vi "Create Progect.vi"(1 "Source DIR":path, 2 "element":string, 3 "selected path":path) -> (0 "Boolean":bool)   [LabVIEW 2019]
panel:
  out "error out":errorcluster
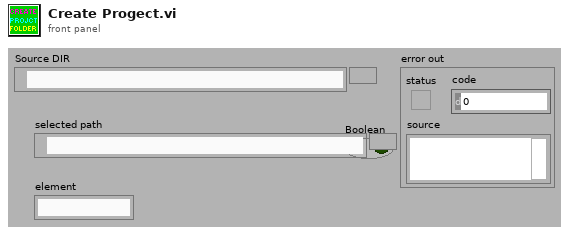
[diagram p1: front panel]
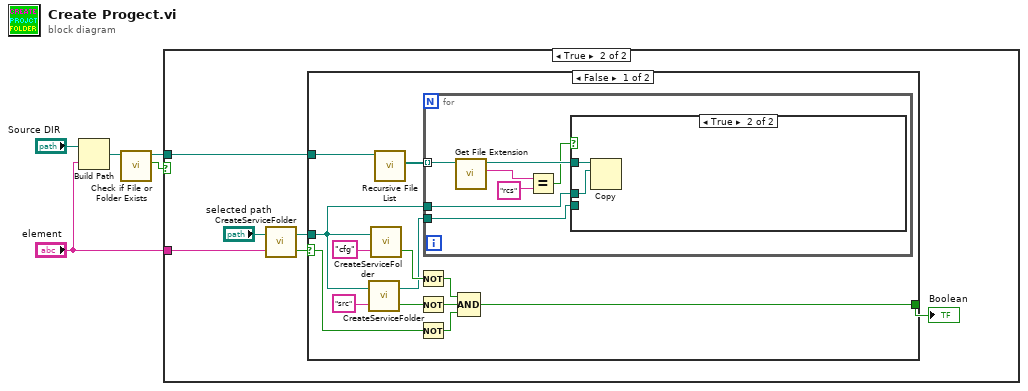
[diagram p0: block diagram]
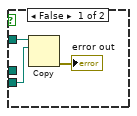
[diagram p3: hidden frame]
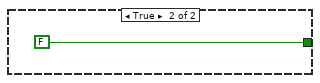
[diagram p4: hidden frame]
diagram:
  n1 = Build Path(base path="Source DIR", name or relative path="element") -> (appended path=w4:path)
  n2 = call <vilib>:"Check if File or Folder Exists.vi"("path"=w4) -> ("file or folder exists?"=w3:bool, "dup path"=w2:path)  [unwired: 8 in, 1 out]
  n3 = case shown="True" w3 {
    tunnel: w2 -> [_ w6]
    tunnel: "element" -> [_ w9]
    frame False {
    }
    frame True {
      n4 = call "CreateServiceFolder.vi"("element"=w9, "selected path"="selected path") -> ("cancelled"=w8:bool, "created path"=w7:path)
      n5 = case shown="False" w8 {
        selector: w8 -> [w21 _]
        tunnel: w7 -> [w12 _]
        tunnel: [w20 FALSE] -> w11
        tunnel: w6 -> [w15 _]
        frame False {
          n6 = call "CreateServiceFolder.vi"("element"="src" ("prompt (Create Folder)"), "selected path"=w12) -> ("cancelled"=w16:bool, "created path"=w13:path)
          n7 = call "CreateServiceFolder.vi"("element"="cfg" ("prompt (Create Folder)"), "selected path"=w12) -> ("cancelled"=w18:bool)  [unwired: 1 out]
          n8 = call <vilib>:"Recursive File List.vi"("Folder Path"=w15) -> ("All Files in Dir"=w14:path[])  [unwired: 6 in, 4 out]
          n9 = Not(x=w18) -> (.not. x?=w24:bool)
          n10 = Not(x=w16) -> (.not. x?=w23:bool)
          n11 = Not(x=w21) -> (.not. x?=w22:bool)
          n12 = for {
            tunnel: w14 -> [w31] mode=indexing
            tunnel: w13 -> [w27]
            tunnel: w12 -> [w26]
            n13 = call <vilib>:"Get File Extension.vi"("file"=w31) -> ("lowercase file extension"=w25:string, "dup file"=w30:path)  [unwired: 6 in, 3 out]
            n14 = Equal?(x=w25, y="rcs" ("lowercase file extension")) -> (x = y?=w28:bool)
            n15 = case shown="True" w28 {
              tunnel: w30 -> [w34 w36]
              tunnel: w27 -> [w33 _]
              tunnel: w26 -> [_ w35]
              frame False {
                n16 = Copy(10:w33, 11:w34) -> (0:→"error out":errorcluster)  [unwired: 3 in, 2 out]
              }
              frame True {
                n17 = Copy(10:w35, 11:w36) -> ()  [unwired: 3 in, 3 out]
              }
            }
          }
          n18 = Compound Arithmetic op=AND(w24, w23, w22) -> (w20:bool)
        }
        frame True {
        }
      }
      "Boolean" <- w11
    }
  }
